vi "Update Cycle Time.vi"(7 "Initialize":bool, 8 "error in (no error)":errorcluster, 10 "T1":u64, 11 "Timing in":cluster{"Max":i32, "Min":i32}) -> (0 "error out":errorcluster, 3 "Timing out":cluster{"Max":i32, "Min":i32})   [LabVIEW 2021, in "CIFCoreCommon.lvlib"]
uses:
  CIFCoreCommon.lvlib
  CIFUtilities/CIFClocks/SubVIs/Add Error.vi
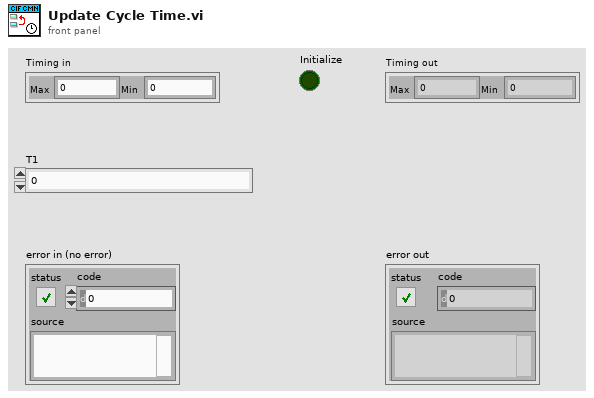
[diagram p1: front panel]
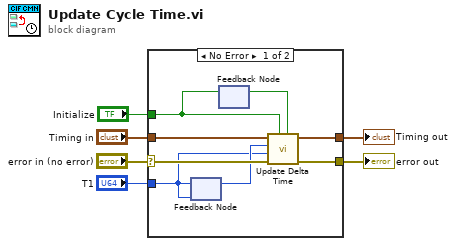
[diagram p0: block diagram]
diagram:
  n1 = case shown="No Error" "error in (no error)" {
    selector: "error in (no error)" -> [w12 w15]
    tunnel: "T1" -> [w9 _]
    tunnel: "Timing in" -> [w14 w16]
    tunnel: [w13 w16] -> w3
    tunnel: [w11 w15] -> w2
    tunnel: "Initialize" -> [w8 _]
    frame No Error {
      n2 = feedback #1(w9) -> (w10:u64)
      n3 = feedback-in #1(w9) -> ()
      n4 = feedback #2() -> (w7:bool)  [unwired: 1 in]
      n5 = feedback-in #2(w8) -> ()
      n6 = call "Update Delta Time.vi"("reinit"=w7, "skip"=w8, "error in (no error)"=w12, "T2"=w9, "T1"=w10, "Timing in"=w14) -> ("error out"=w11:errorcluster, "Timing out"=w13:cluster{"Max":i32, "Min":i32})  [unwired: 4 in]
    }
    frame Error {
    }
  }
  "Timing out" <- w3
  "error out" <- w2
